vi "StopSignal-TestMain2.vi"() -> ()   [LabVIEW 2017, in "StopSignal.lvlib"]
uses:
  StopSignal.lvlib
panel:
  out "number":i32
  out "timestamp 3":timestamp
  out "timestamp 2":timestamp
  out "timestamp 1":timestamp
  out "Array 4":timestamp[](array[timestamp])
  in  "2":bool
  in  "1":bool
  in  "0":bool
  out "Stop? 3":bool
  out "Stop? 2":bool
  out "Stop? 1":bool
  out "Array 3":string[](array[string])
  in  "Array 2":bool[](array[boolean])
  out "Array":bool[](array[boolean])
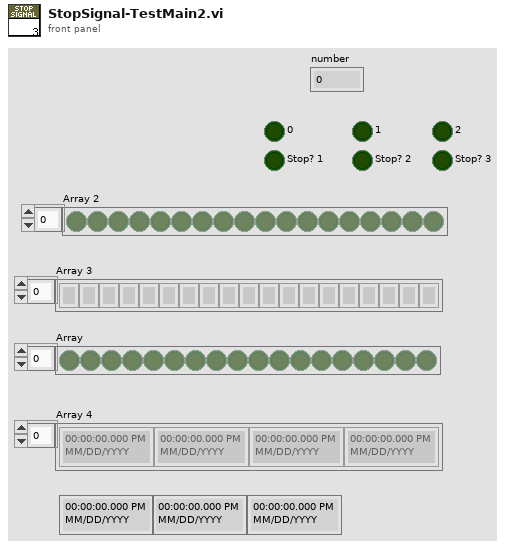
[diagram p1: front panel]
types:
  T1 = typedef "StopSignal.lvlib/StopSignal.ctl" = refnum<k1>
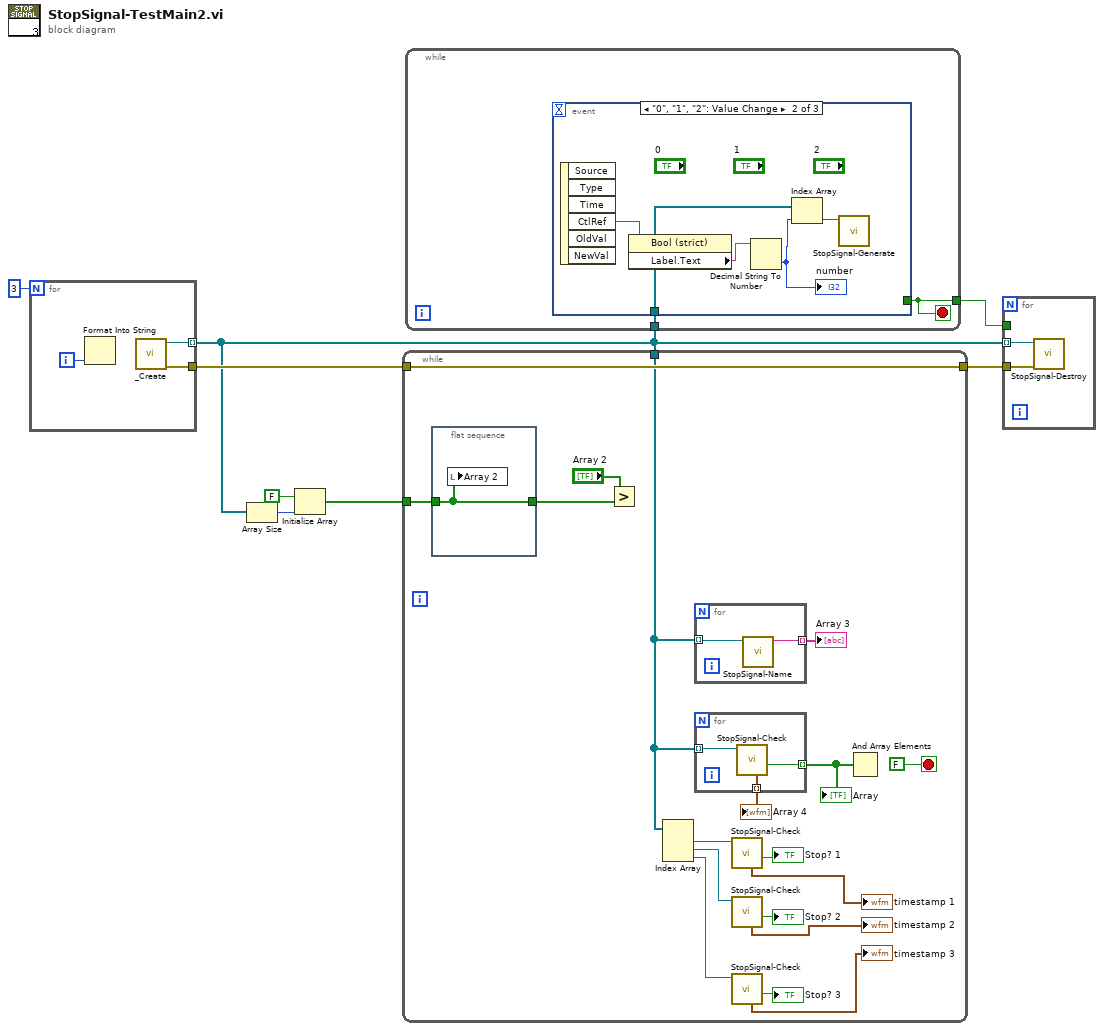
[diagram p0: block diagram]
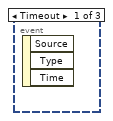
[diagram p2: hidden frame]
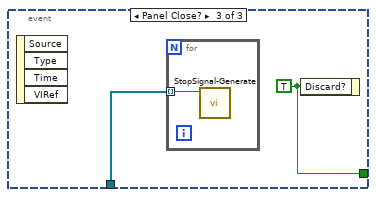
[diagram p3: hidden frame]
diagram:
  n1 = for {
    N: 3 -> [_]
    tunnel: [w11] -> w3 mode=indexing
    tunnel: [w10] -> w4
    i -> [w9]
    n2 = Format Into String(w9) -> ()  [unwired: 3 in, 2 out]
    n3 = call "_Create.vi"() -> ("error out"=w10:errorcluster, "StopSignal"=w11:T1)  [unwired: 10 in]
  }
  n4 = Array Size(array=w3) -> (size(s)=w7:i32)
  n5 = Initialize Array(FALSE, w7) -> (w2:bool[])
  n6 = while {
    tunnel: w3 -> [w25]
    tunnel: [w27] -> w5
    tunnel: w4 -> [w27]
    tunnel: w2 -> [w17]
    stop <- FALSE stop-if-true
    n7 = flat-sequence {
      tunnel: [w35] -> w29
      tunnel: w17 -> [w35]
      frame #0 {
        n8 = local write "Array 2"(w35) -> ()
      }
    }
    n9 = Greater?(x="Array 2", y=w29) -> ()  [unwired: 1 out]
    n10 = Index Array(array=w25) -> (element #1=w24:T1, element #2=w23:T1, element #3=w22:T1)  [unwired: 3 in]
    n11 = for {
      tunnel: w25 -> [w31] mode=indexing
      tunnel: [w30] -> w26 mode=indexing
      n12 = call "StopSignal-Name.vi"("StopSignal"=w31) -> ("name"=w30:string)  [unwired: 9 in, 1 out]
    }
    "Array 3" <- w26
    n13 = for {
      tunnel: [w34] -> w28 mode=indexing
      tunnel: w25 -> [w33] mode=indexing
      tunnel: [w32] -> w16 mode=indexing
      n14 = call "StopSignal-Check.vi"("StopSignal"=w33) -> ("Stop?"=w34:bool, "timestamp"=w32:timestamp)  [unwired: 6 in, 3 out]
    }
    "Array" <- w28
    "Array 4" <- w16
    n15 = call "StopSignal-Check.vi"("StopSignal"=w24) -> ("Stop?"=→"Stop? 1":bool, "timestamp"=→"timestamp 1":timestamp)  [unwired: 6 in, 3 out]
    n16 = call "StopSignal-Check.vi"("StopSignal"=w23) -> ("Stop?"=→"Stop? 2":bool, "timestamp"=→"timestamp 2":timestamp)  [unwired: 6 in, 3 out]
    n17 = call "StopSignal-Check.vi"("StopSignal"=w22) -> ("Stop?"=→"Stop? 3":bool, "timestamp"=→"timestamp 3":timestamp)  [unwired: 6 in, 3 out]
    n18 = And Array Elements(Boolean array=w28) -> ()  [unwired: 1 out]
  }
  n19 = while {
    tunnel: w3 -> [w37]
    tunnel: [w36] -> w1
    stop <- w36 stop-if-true
    n20 = event shown="[1] \"0\", \"1\", \"2\": Value Change" {
      selector: _ -> [_ _ _]
      dyn-events: _ -> [_ _ _]
      timeout: _ -> [_ _ _]
      tunnel: w37 -> [_ w42 w44]
      tunnel: [_ _ w43] -> w36
      event Timeout {
        n21 = event-data() -> ()  [unwired: 1 in, 3 out]
      }
      event "0", "1", "2": Value Change {
        n22 = event-data() -> ("CtlRef"=w40:refnum<vi>)  [unwired: 1 in, 5 out]
        n23 = property class="Bool (strict)"(reference=w40) -> ("Label.Text"=w39:string)  [unwired: 1 in, 2 out]
        n24 = Decimal String To Number(string=w39) -> (number=w38:i32)  [unwired: 2 in, 1 out]
        "number" <- w38
        n25 = Index Array(array=w42, index=w38) -> (element=w41:T1)
        n26 = call "StopSignal-Generate.vi"("StopSignal"=w41) -> ()  [unwired: 9 in, 2 out]
      }
      event Panel Close? {
        w43 = TRUE ("Discard?")
        n27 = event-data() -> ()  [unwired: 1 in, 4 out]
        n28 = for {
          tunnel: w44 -> [w45] mode=indexing
          n29 = call "StopSignal-Generate.vi"("StopSignal"=w45) -> ()  [unwired: 9 in, 2 out]
        }
        n30 = event-data("Discard?"=w43) -> ()  [unwired: 1 in, 1 out]
      }
    }
  }
  n31 = for {
    tunnel: w3 -> [w47] mode=indexing
    tunnel: w5 -> [w46]
    tunnel: w1 -> [_]
    n32 = call "StopSignal-Destroy.vi"("error in (no error)"=w46, "StopSignal"=w47) -> ()  [unwired: 9 in, 1 out]
  }
